vi "Triggering DIO Pattern.vi"(8 "error in (no error)":errorcluster, 10 "pattern":string, 11 "MicroDAQ.lvlib:Analog Input.lvclass":refnum<class "Analog Input.lvclass">) -> (0 "error out":errorcluster, 3 "MicroDAQ.lvlib:Analog Input.lvclass out":refnum<class "Analog Input.lvclass">)   [LabVIEW 2009, in "MicroDAQ.lvlib" / "Analog Input.lvclass"]
doc: "This function configures DIO pattern trigger for AO/AI scan operation. The pattern argument must contains eight characters string with 'x', '1' or '0' defining desired DIO1...8 state. The 'x' character indicates that DIO is state is ignored, while 0 and 1 indicated low and high state respectively. DIO pattern defines DIO state in the following order DIO1, DIO2, DIO3, DIO4, DIO5, DIO6, DIO7, DIO8 e.g. pattern '11xxxxxx' is related to DIO1 and DIO2 state."
uses:
  <instrlib>/MicroDAQ/Channel/Analog Input/Analog Input.lvclass
  <instrlib>/MicroDAQ/Tools/Trigger type.ctl
  <instrlib>/MicroDAQ/Channel/Channel.lvclass
  <instrlib>/MicroDAQ/Mlink library wraper/mlink.lvlib
  <instrlib>/MicroDAQ/MicroDAQ.lvlib
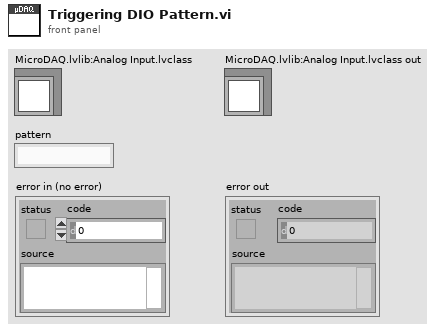
[diagram p1: front panel]
types:
  T1 = typedef "MicroDAQ.lvlib/Trigger type.ctl" = enum8{"Analog output", "Analog input"}
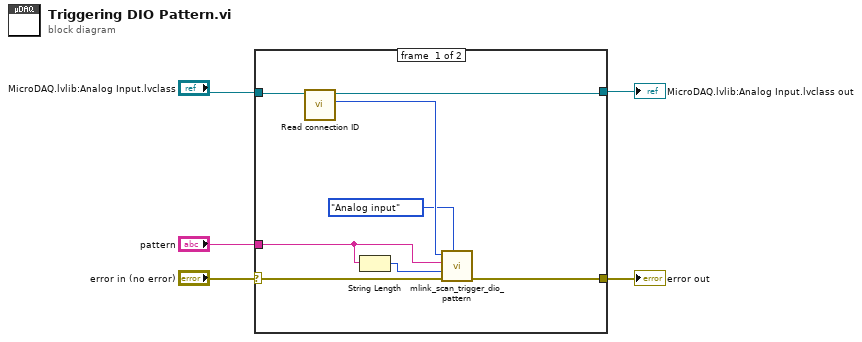
[diagram p0: block diagram]
diagram:
  n1 = case shown="No Error" "error in (no error)" {
    selector: "error in (no error)" -> [w11 w14]
    tunnel: [w10 w14] -> w4
    tunnel: [w12 w15] -> w3
    tunnel: "MicroDAQ.lvlib:Analog Input.lvclass" -> [w13 w15]
    tunnel: "pattern" -> [w7 _]
    frame #0 {
      n2 = call <instrlib>:"Read connection ID.vi"("Task in"=w13) -> ("connection ID"=w9:i32, "Task out"=w12:refnum<class "Analog Input.lvclass">)  [unwired: 9 in]
      n3 = String Length(string=w7) -> (length=w6:i32)
      n4 = call <instrlib>:"mlink_scan_trigger_dio_pattern.vi"("trigger type"=Trigger_type."Analog input", "error in (no error)"=w11, "len"=w6, "pattern"=w7, "connection ID"=w9) -> ("error out"=w10:errorcluster)  [unwired: 5 in, 1 out]
    }
    frame #1 {
    }
  }
  "error out" <- w4
  "MicroDAQ.lvlib:Analog Input.lvclass out" <- w3
